vi "抽样与分割.vi"(8 "采样数":i32, 9 "采样率":i32[](array[numeric])=[32000, 32000, 32000, 32000, 32000, 32000, 80000, 80000], 10 "6133队列":refnum<queue>, 11 "DataQRef":refnum<queue>) -> ()   [LabVIEW 2014]
panel:
  in  "发送次数":i32=160
  out "每通道发送的数据量":i32[](array[numeric])
  in  "读取次数":dbl=1.0
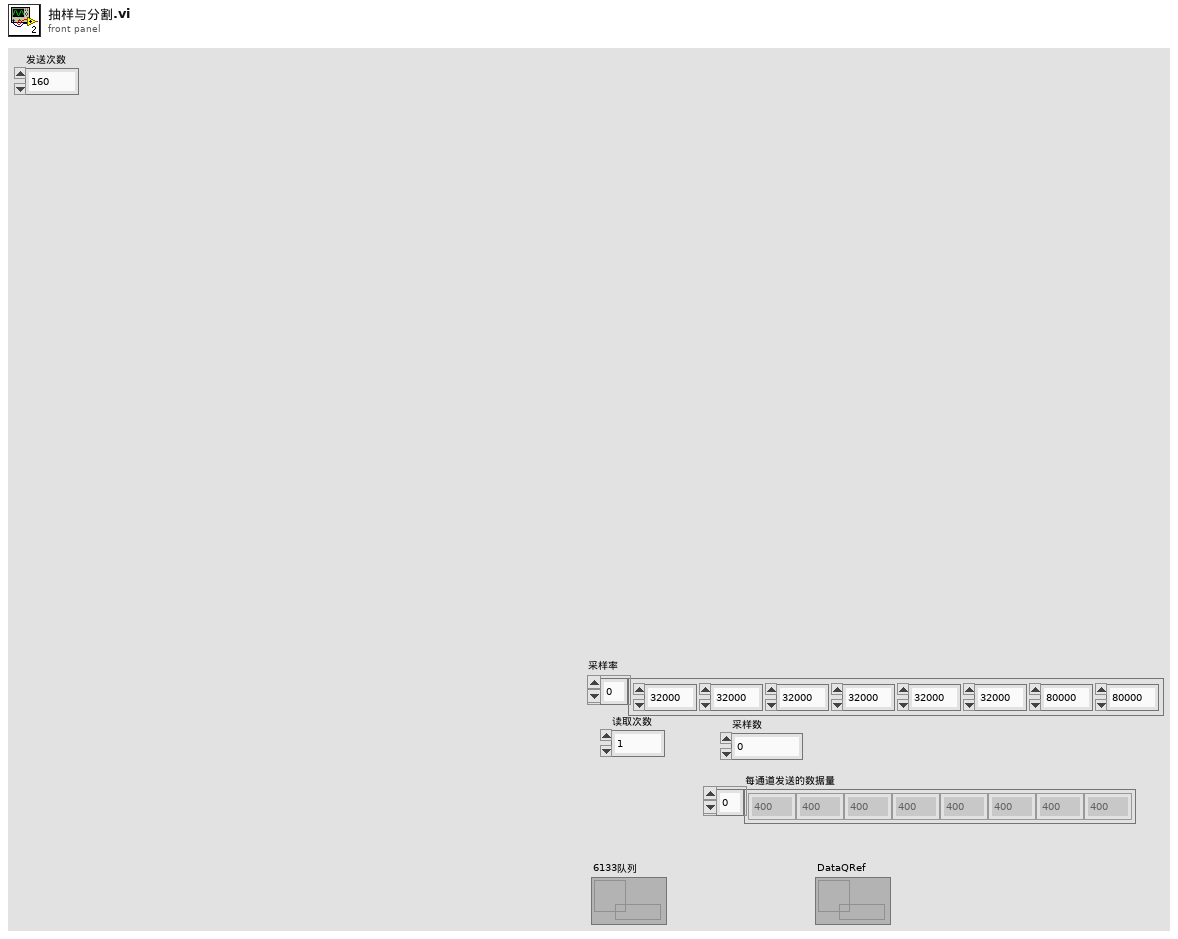
[diagram p1: front panel]
types:
  T1 = cluster{"时间":timestamp, "声发射":sgl[], "电涡流1":sgl[], "电涡流2":sgl[], "电涡流3":sgl[], "电涡流4":sgl[], "电涡流5":sgl[], "加速度1":sgl[], "加速度2":sgl[]}
  T2 = cluster{"设备名":string, "时间":timestamp, "数据":sgl[][]}
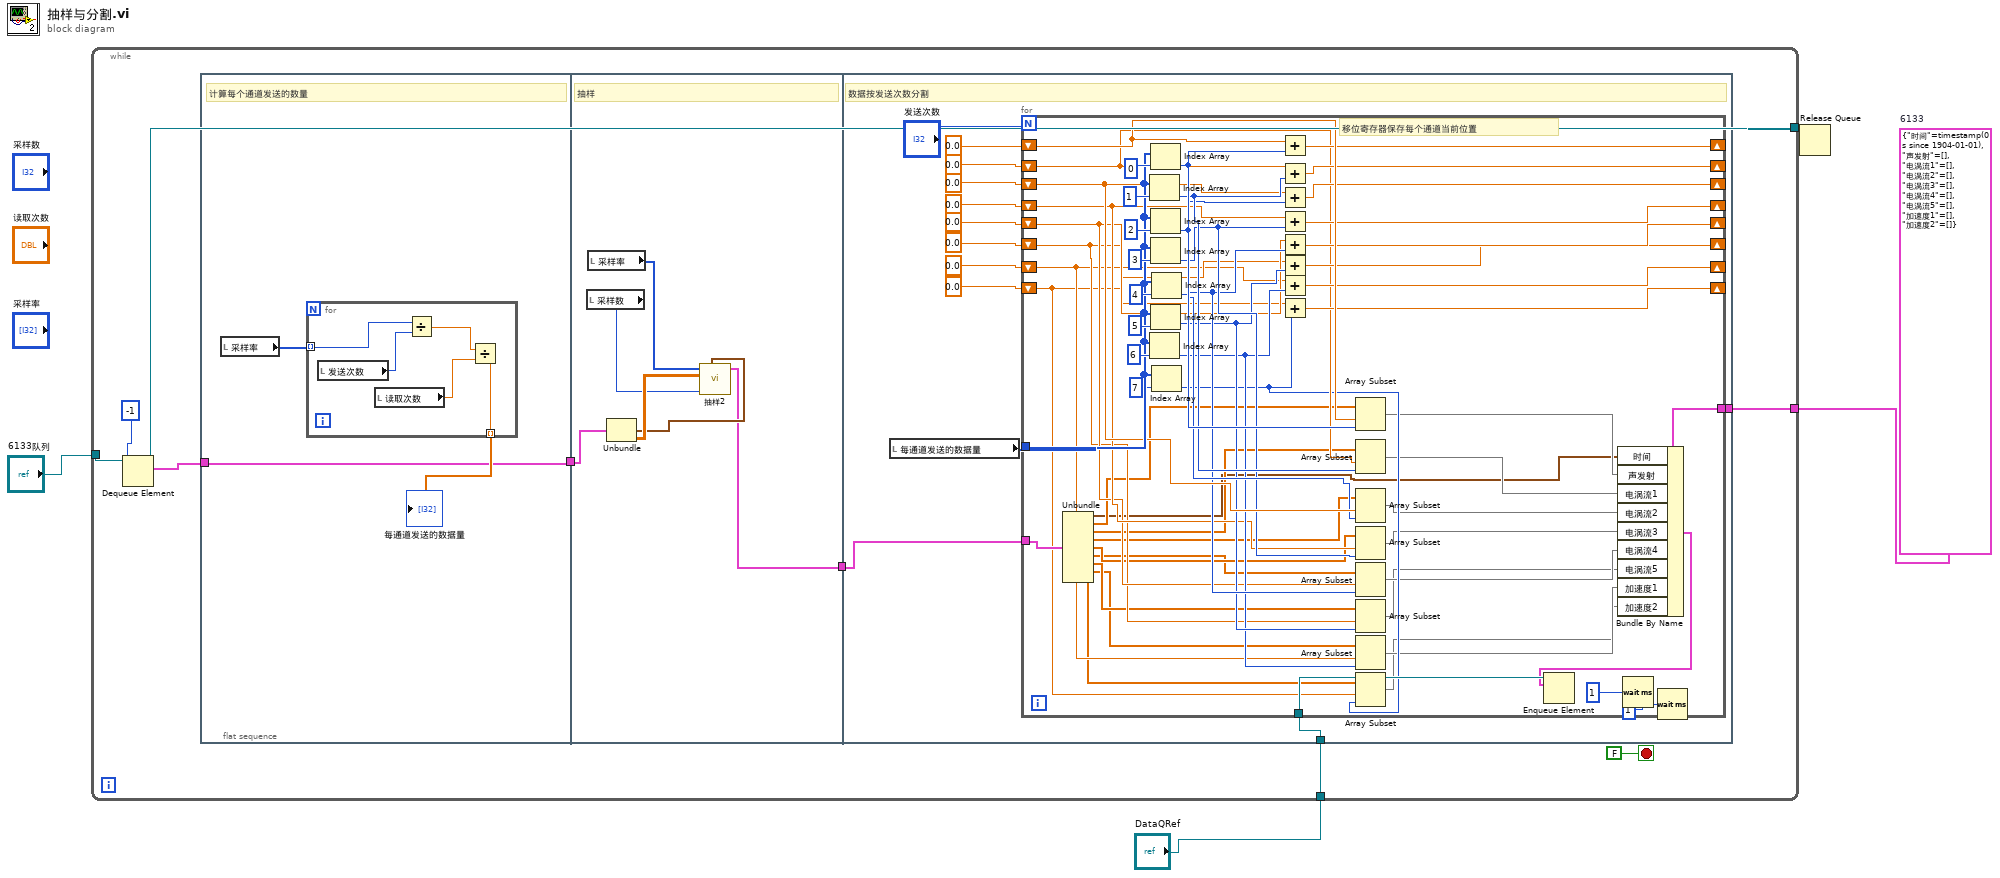
[diagram p0: block diagram]
diagram:
  w2 = T1 {"时间"=timestamp(0 s since 1904-01-01), "声发射"=[], "电涡流1"=[], "电涡流2"=[], "电涡流3"=[], "电涡流4"=[], "电涡流5"=[], "加速度1"=[], "加速度2"=[]}  # 6133
  n1 = while "While循环" {
    tunnel: "6133队列" -> [w13]
    tunnel: [w12] -> w4
    tunnel: "DataQRef" -> [w10]
    tunnel: w2 -> [w5]
    stop <- FALSE stop-if-true
    n2 = Dequeue Element(queue=w13, timeout in ms (-1)=-1 ("超时毫秒(-1)")) -> (queue out=w12:refnum<queue>, element=w9:T2)  [unwired: 1 in, 2 out]
    n3 = flat-sequence "平铺式顺序结构" {
      tunnel: [w14] -> w8
      tunnel: w9 -> [w14]
      tunnel: w8 -> [w27]
      tunnel: [w22] -> w7
      tunnel: w10 -> [w29]
      tunnel: w7 -> [w30]
      tunnel: w5 -> [w28]
      frame #0 {
        # "计算每个通道发送的数量"
        n4 = local read "采样率"() -> (w16:i32[])
        n5 = for "For循环" {
          tunnel: w16 -> [w18] mode=indexing
          tunnel: [w17] -> w15 mode=indexing
          n6 = local read "发送次数"() -> (w19:i32)
          n7 = local read "读取次数"() -> (w21:dbl)
          n8 = Divide(x=w18, y=w19) -> (x/y=w20:dbl)
          n9 = Divide(x=w20, y=w21) -> (x/y=w17:dbl)
        }
        "每通道发送的数据量" <- w15
      }
      frame #1 {
        # "抽样"
        n10 = local read "采样数"() -> (w24:i32)
        n11 = local read "采样率"() -> (w26:i32[])
        n12 = Unbundle(w27) -> ("时间"=w23:timestamp, "数据"=w25:sgl[][])  [unwired: 1 out]
        n13 = call "抽样2.vi"("时间标识"=w23, "采样数"=w24, "采集数据"=w25, "采样率"=w26) -> ("6133"=w22:T1)  [unwired: 6 in, 1 out]
      }
      frame #2 {
        # "数据按发送次数分割"
        n14 = local read "每通道发送的数据量"() -> (w40:i32[])
        n15 = for {
          N: "发送次数" -> [_]
          shift-right: [w95] -> _
          shift-left: 0.0 ("元素") -> [w96]
          tunnel: w30 -> [w92]
          tunnel: w40 -> [w76]
          tunnel: w29 -> [w94]
          shift-right: [w89] -> _
          shift-left: 0.0 ("元素") -> [w73]
          shift-right: [w88] -> _
          shift-left: 0.0 ("元素") -> [w72]
          shift-right: [w87] -> _
          shift-left: 0.0 ("元素") -> [w65]
          shift-right: [w86] -> _
          shift-left: 0.0 ("元素") -> [w64]
          shift-right: [w85] -> _
          shift-left: 0.0 ("元素") -> [w63]
          shift-right: [w84] -> _
          shift-left: 0.0 ("元素") -> [w62]
          shift-right: [w83] -> _
          shift-left: 0.0 ("元素") -> [w61]
          tunnel: w28 -> [w60]
          # "移位寄存器保存每个通道当前位置"
          n16 = Unbundle(w92) -> ("时间"=w48:timestamp, "声发射"=w50:sgl[], "电涡流1"=w49:sgl[], "电涡流2"=w47:sgl[], "电涡流3"=w46:sgl[], "电涡流4"=w45:sgl[], "电涡流5"=w44:sgl[], "加速度1"=w43:sgl[], "加速度2"=w42:sgl[])
          n17 = Index Array(array=w76, index=1 ("索引")) -> (element=w74:i32)
          n18 = Index Array(array=w76, index=6 ("索引")) -> (element=w67:i32)
          n19 = Index Array(array=w76, index=0 ("索引")) -> (element=w90:i32)
          n20 = Index Array(array=w76, index=2 ("索引")) -> (element=w71:i32)
          n21 = Index Array(array=w76, index=3 ("索引")) -> (element=w70:i32)
          n22 = Index Array(array=w76, index=5 ("索引")) -> (element=w68:i32)
          n23 = Index Array(array=w76, index=4 ("索引")) -> (element=w69:i32)
          n24 = Index Array(array=w76, index=7 ("索引")) -> (element=w66:i32)
          n25 = Add(x=w96, y=w90) -> (x+y=w95:dbl)
          n26 = Add(x=w73, y=w74) -> (x+y=w89:dbl)
          n27 = Add(x=w72, y=w71) -> (x+y=w88:dbl)
          n28 = Add(x=w65, y=w70) -> (x+y=w87:dbl)
          n29 = Add(x=w64, y=w69) -> (x+y=w86:dbl)
          n30 = Add(x=w63, y=w68) -> (x+y=w85:dbl)
          n31 = Add(x=w62, y=w67) -> (x+y=w84:dbl)
          n32 = Add(x=w61, y=w66) -> (x+y=w83:dbl)
          n33 = Array Subset ("数组子集")(array=w50, index=w96, length=w90) -> (w58:sgl[])
          n34 = Array Subset ("数组子集")(array=w49, index=w73, length=w74) -> (w57:sgl[])
          n35 = Array Subset ("数组子集")(array=w47, index=w72, length=w71) -> (w56:sgl[])
          n36 = Array Subset ("数组子集")(array=w46, index=w65, length=w70) -> (w55:sgl[])
          n37 = Array Subset ("数组子集")(array=w45, index=w64, length=w69) -> (w54:sgl[])
          n38 = Array Subset ("数组子集")(array=w44, index=w63, length=w68) -> (w53:sgl[])
          n39 = Array Subset ("数组子集")(array=w43, index=w62, length=w67) -> (w52:sgl[])
          n40 = Array Subset ("数组子集")(array=w42, index=w61, length=w66) -> (w51:sgl[])
          n41 = Bundle By Name(cluster=w60, "时间"=w48, "声发射"=w58, "电涡流1"=w57, "电涡流2"=w56, "电涡流3"=w55, "电涡流4"=w54, "电涡流5"=w53, "加速度1"=w52, "加速度2"=w51) -> (w59:T1)
          n42 = Enqueue Element(queue=w94, element=w59) -> ()  [unwired: 2 in, 3 out]
          n43 = Wait (ms)(milliseconds to wait=u32 1 ("等待时间（毫秒）")) -> ()  [unwired: 1 out]
        }
        n44 = Wait (ms)(milliseconds to wait=u32 1 ("等待时间（毫秒）")) -> ()  [unwired: 1 out]
      }
    }
  }
  n45 = Release Queue(queue=w4) -> ()  [unwired: 2 in, 3 out]
